vi "test Diff Configuration (Add Port).vi"(8 "error in":errorcluster, 11 "TestCase in":refnum<class "Refresh.lvclass">) -> (0 "error out":errorcluster, 3 "TestCase out":refnum<class "Refresh.lvclass">)   [LabVIEW 2020, in "Refresh.lvclass"]
uses:
  Refresh.lvclass
  <vilib>/addons/_JKI Toolkits/VI Tester/TestCase.llb/TestCase.lvclass
  System Explorer/Implementation/System Explorer/Refresh/Refresh.lvlib
  Shared/Parameter Definition.ctl
  Shared/Address.ctl
  Shared/Terminal Endpoint.ctl
  Shared/Message Type.ctl
  Shared/Message Definition.ctl
  Shared/BIU Configuration.ctl
  System Explorer/Implementation/System Explorer/Refresh/Symbols.ctl
  System Explorer/Implementation/System Explorer/Refresh/Change Type.ctl
  System Explorer/Implementation/System Explorer/Refresh/MCL Row.ctl
  Shared/Minor Frame Definition.ctl
  Shared/Major Frame Definition.ctl
  Shared/Acyclic Frame Definition.ctl
  C:/Program Files (x86)/National Instruments/LabVIEW 2020/vi.lib/addons/_JKI Toolkits/VI Tester/TestCase.llb/TestCase.lvclass
panel:
  out "Multicolumn Listbox":i32(listbox)=-1
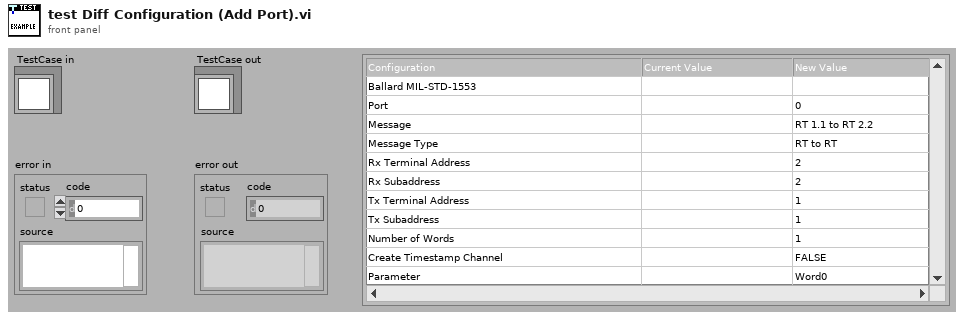
[diagram p1: front panel]
types:
  T1 = typedef "Message Definition.ctl" = cluster{"name":string, "message type":T2, "endpoint Tx":T3, "endpoint Rx":T3, "create timestamp channel":bool, "mode code":u16, "number of words":u16, "parameters":cluster{"name":string, "default value":dbl, "unit":string, "parameter definition":T5}[]}
  T2 = typedef "Message Type.ctl" = string
  T3 = typedef "Terminal Endpoint.ctl" = cluster{"terminal address":T4, "subaddress":T4}
  T4 = typedef "Address.ctl" = u16
  T5 = typedef "Parameter Definition.ctl" = cluster{"start index":i32, "size (bits)":i32, "encoding":enum16{"BNR", "BCD", "Discrete"}, "signed":bool, "multiplier":dbl, "offset":dbl}
  T6 = typedef "BIU Configuration.ctl" = cluster{"HW channel":u16, "terminal addresses":T4[], "terminal names":string[], "major frames":T7[], "minor frames":T8[], "acyclic frames":T9[], "messages":T1[]}
  T7 = typedef "Major Frame Definition.ctl" = cluster{"name":string, "minor frames":string[]}
  T8 = typedef "Minor Frame Definition.ctl" = cluster{"name":string, "messages":string[]}
  T9 = typedef "Acyclic Frame Definition.ctl" = cluster{"name":string, "messages":string[]}
  T10 = typedef "AIM MIL-STD-1553 System Explorer.lvlib/Implementation.lvlib/Refresh.lvlib/MCL Row.ctl" = cluster{"change type":T11, "item symbol":T12, "item names":string[]}
  T11 = typedef "AIM MIL-STD-1553 System Explorer.lvlib/Implementation.lvlib/Refresh.lvlib/Change Type.ctl" = enum16{"No change", "Modify", "Add", "Remove"}
  T12 = typedef "AIM MIL-STD-1553 System Explorer.lvlib/Implementation.lvlib/Refresh.lvlib/Symbols.ctl" = enum16{"Blank", "MIL-STD-1553", "Port", "Remote Terminal", "Subaddress", "Bus Controller", "Acyclic Frame", "Mode Code", "Message", "Parameter", "Item"}
  T13 = typedef "imagedata.ctl" = cluster{"image type":i32, "image depth":i32, "image":u8[], "mask":u8[], "colors":u32[], "Rectangle":cluster{"left":i16, "top":i16, "right":i16, "bottom":i16}}
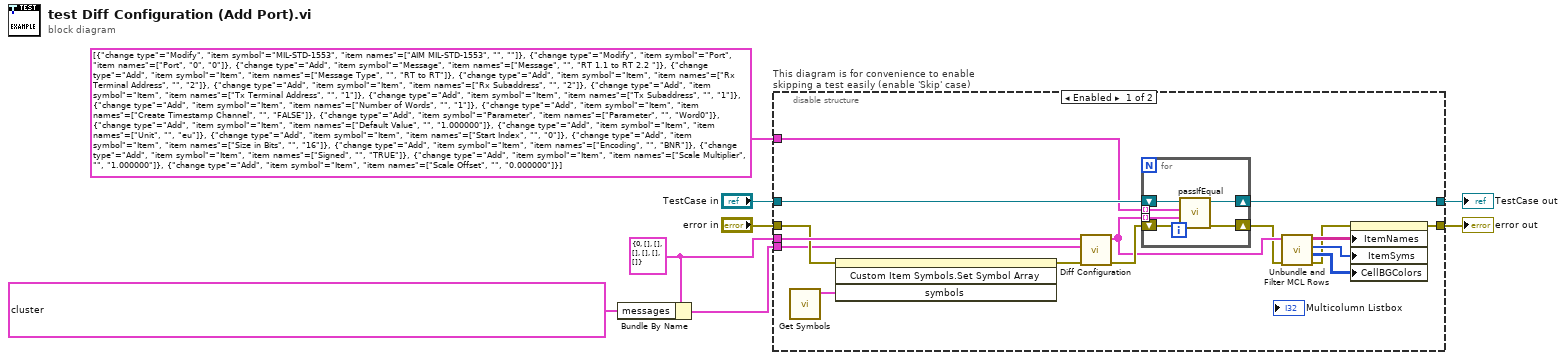
[diagram p0: block diagram]
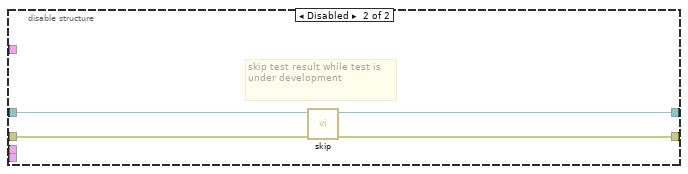
[diagram p2: hidden frame]
diagram:
  w1 = T6 {"HW channel"=0, "terminal addresses"=[], "terminal names"=[], "major frames"=[], "minor frames"=[], "acyclic frames"=[], "messages"=[]} ("1553 channel")
  n1 = Bundle By Name(cluster=w1, "messages"=T1[] [{"name"="RT 1.1 to RT 2.2 ", "message type"="RT to RT", "endpoint Tx"={"terminal address"=1, "subaddress"=1}, "endpoint Rx"={"terminal address"=2, "subaddress"=2}, "create timestamp channel"=FALSE, "mode code"=0, "number of words"=1, "parameters"=[{"name"="Word0", "default value"=1.0, "unit"="eu", "parameter definition"={"start index"=0, "size (bits)"=16, "encoding"=enum."BNR", "signed"=TRUE, "multiplier"=1.0, "offset"=0.0}}]}]) -> (w3:T6)
  n2 = disable-structure "This diagram is for convenience to enable skipping a test easily (enable 'Skip' case)" shown="Enabled" {
    disable-tunnel: "TestCase in" -> [w24 w34]
    disable-tunnel: [w23 w32] -> w5
    disable-tunnel: [w13 w33] -> w7
    disable-tunnel: "error in" -> [w11 w31]
    disable-tunnel: w1 -> [w22 _]
    disable-tunnel: w3 -> [w9 _]
    disable-tunnel: T10[] [{"change type"=enum."Modify", "item symbol"=enum."MIL-STD-1553", "item names"=["AIM MIL-STD-1553", "", ""]}, {"change type"=enum."Modify", "item symbol"=enum."Port", "item names"=["Port", "0", "0"]}, {"change type"=enum."Add", "item symbol"=enum."Message", "item names"=["Message", "", "RT 1.1 to RT 2.2 "]}, {"change type"=enum."Add", "item symbol"=enum."Item", "item names"=["Message Type", "", "RT to RT"]}, {"change type"=enum."Add", "item symbol"=enum."Item", "item names"=["Rx Terminal Address", "", "2"]}, {"change type"=enum."Add", "item symbol"=enum."Item", "item names"=["Rx Subaddress", "", "2"]}, {"change type"=enum."Add", "item symbol"=enum."Item", "item names"=["Tx Terminal Address", "", "1"]}, {"change type"=enum."Add", "item symbol"=enum."Item", "item names"=["Tx Subaddress", "", "1"]}, {"change type"=enum."Add", "item symbol"=enum."Item", "item names"=["Number of Words", "", "1"]}, {"change type"=enum."Add", "item symbol"=enum."Item", "item names"=["Create Timestamp Channel", "", "FALSE"]}, {"change type"=enum."Add", "item symbol"=enum."Parameter", "item names"=["Parameter", "", "Word0"]}, {"change type"=enum."Add", "item symbol"=enum."Item", "item names"=["Default Value", "", "1.000000"]}, {"change type"=enum."Add", "item symbol"=enum."Item", "item names"=["Unit", "", "eu"]}, {"change type"=enum."Add", "item symbol"=enum."Item", "item names"=["Start Index", "", "0"]}, {"change type"=enum."Add", "item symbol"=enum."Item", "item names"=["Size in Bits", "", "16"]}, {"change type"=enum."Add", "item symbol"=enum."Item", "item names"=["Encoding", "", "BNR"]}, {"change type"=enum."Add", "item symbol"=enum."Item", "item names"=["Signed", "", "TRUE"]}, {"change type"=enum."Add", "item symbol"=enum."Item", "item names"=["Scale Multiplier", "", "1.000000"]}, {"change type"=enum."Add", "item symbol"=enum."Item", "item names"=["Scale Offset", "", "0.000000"]}] ("configuration diff") -> [w21 _]
    frame Enabled {
      n3 = call "Get Symbols.vi"() -> ("MIL-STD-1553 symbols"=w12:T13[])  [unwired: 11 in]
      n4 = invoke on="Multicolumn Listbox" class="MCListbox (strict)" method="Custom Item Symbols.Set Symbol Array"(error in=w11, "symbols"=w12) -> (error out=w10:errorcluster)  [unwired: 2 in, 3 out]
      n5 = call "Diff Configuration.vi"("error in"=w10, "configuration new"=w9, "configuration old"=w22) -> ("error out"=w20:errorcluster, "configuration diff"=w19:T10[])  [unwired: 7 in]
      n6 = for {
        tunnel: w21 -> [w28] mode=indexing
        tunnel: w19 -> [w26] mode=indexing
        shift-right: [w29] -> w23
        shift-left: w24 -> [w30]
        shift-right: [w25] -> w15
        shift-left: w20 -> [w27]
        n7 = call-dynamic "passIfEqual.vi"("error in (no error)"=w27, "y"=w26, "x"=w28, "TestCase in"=w30) -> ("error out"=w25:errorcluster, "TestCase out"=w29:refnum<class "Refresh.lvclass">)  [unwired: 6 in]
      }
      n8 = call "Unbundle and Filter MCL Rows.vi"("error in"=w15, "refresh items"=w19) -> ("error out"=w14:errorcluster, "background colors"=w18:u32[][], "item symbols"=w17:T12[], "item names"=w16:string[][])  [unwired: 6 in]
      n9 = property on="Multicolumn Listbox" class="MCListbox (strict)"(error in=w14, "ItemNames"=w16, "ItemSyms"=w17, "CellBGColors"=w18) -> (error out=w13:errorcluster)  [unwired: 1 in, 1 out]
    }
    frame Disabled {
      # "skip test result while test is under development"
      n10 = call <vilib>:"skip.vi"("error in (no error)"=w31, "TestCase in"=w34) -> ("error out"=w33:errorcluster, "TestCase out"=w32:refnum<class "Refresh.lvclass">)  [unwired: 8 in]
    }
  }
  "error out" <- w7
  "TestCase out" <- w5
